vi "Get OS.vi"(8 "error in (no error)":errorcluster, 11 "RT Management in":refnum<class "RT Management.lvclass">) -> (0 "error out":errorcluster, 1 "Operating System Architecture":string, 2 "Operating System":T1, 3 "RT Management out":refnum<class "RT Management.lvclass">)   [LabVIEW 2016, in "RT Management.lvlib" / "RT Management.lvclass"]
doc: "Returns the OS of the RT target. The possible values for the \"Operating System\" enum are: Unknown, VxWorks, PharLap, Linux-ARM, and Linux-x64.\n\nThe \"Operating System Architecture\" strings returns the exact string that the System Configuration API returns, even in the case of Unknown."
uses:
  RT Management.lvclass
  Controls/Operating system.ctl
  RT Management.lvclass/RT Management.ctl
  Get Operating system.vi
  Get Operating System Architecture.vi
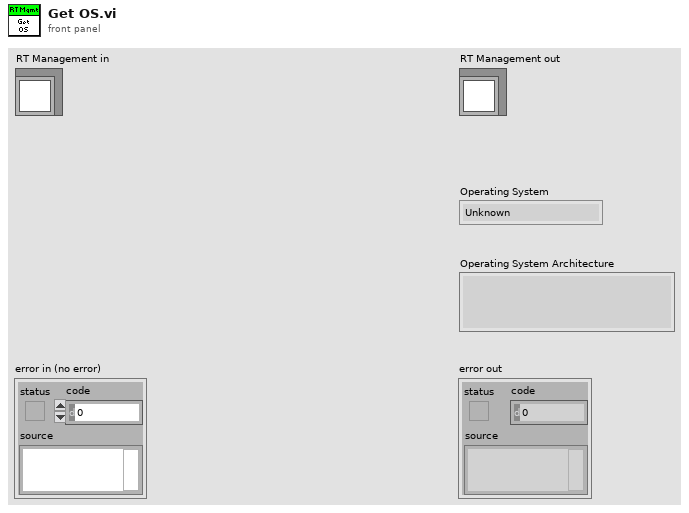
[diagram p1: front panel]
types:
  T1 = typedef "RT Management.lvlib/RT Management.lvclass/Operating system.ctl" = enum16{"Unknown", "VxWorks", "PharLap", "Linux-ARM", "Linux-x64"}
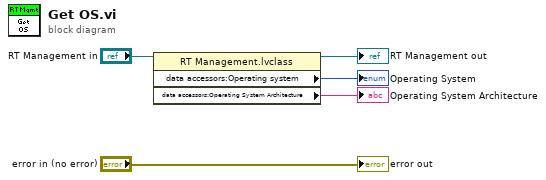
[diagram p0: block diagram]
diagram:
  n1 = property class="RT Management.lvclass"(reference="RT Management in") -> (reference out=→"RT Management out":refnum<class "RT Management.lvclass">, "data accessors:Operating system"=→"Operating System":T1, "data accessors:Operating System Architecture"=→"Operating System Architecture":string)  [unwired: 1 in, 1 out]
  "error out" <- "error in (no error)"
